vi "Drive Code.vi"() -> ()   [LabVIEW 2020]
uses:
  Team Code/Robot Global Data.vi
panel:
  out "LoopTime (ms)":u32
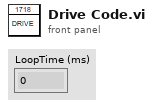
[diagram p1: front panel]
types:
  T1 = typedef "PiConfig.ctl" = cluster{"swerveModules":cluster{"leftFront":T2, "rightFront":T2, "leftRear":T2, "rightRear":T2}, "offsets":cluster{"leftFrontAngleOffset":dbl, "leftRearAngleOffset":dbl, "rightFrontAngleOffset":dbl, "rightRearAngleOffset":dbl}, "limits":cluster{"maxVelocity":dbl, "maxOverdriveVelocity":dbl, "maxAcceleration":dbl, "maxPickupVelocity":dbl, "maxClimbArmVelocity":dbl}, "speeds":cluster{"intakeSuckSpeed":dbl, "intakeSpitSpeed":dbl, "indexerSuckSpeed":dbl, "indexerSpitSpeed":dbl, "indexerShootSpeed":dbl, "indexerBumpBackSpeed":dbl, "shooterSpinupSpeed":dbl, "kickupSpinupSpeed":dbl, "shooterLowShootSpeed":dbl, "shooterHighShootSpeed":dbl, "shooterPadSpeed":dbl, "shooterWallSpeed":dbl}, "positions":cluster{"intakeStarting":dbl, "intakeStow":dbl, "intakeSuck":dbl, "armPounce":dbl, "armStow":dbl, "armUp":dbl, "winchPounce":dbl, "winchOut":dbl, "winchStow":dbl, "intakeSpit":dbl, "winchBarEngage":dbl, "winchBottomClimb":dbl, "hoodHighShoot":dbl, "armClearHooks":dbl, "winchClearHooks":dbl, "armLiftNextBar":dbl, "winchEngageHooksNextBar":dbl, "winchEngagePassive":dbl, "winchTraversalClimb":dbl, "hoodPadShoot":dbl, "turretPadShoot":dbl, "hoodWallShoot":dbl, "turretWallShoot":dbl, "winchRobotOffBar":dbl, "winchSettleClimb":dbl}, "inversions":cluster{"rightShooter":bool, "leftShooter":bool}}
  T2 = typedef "Swerve Module Parameters.ctl" = cluster{"driveCANID":dbl, "angleCANID":i32, "canCoderCANID":dbl, "moduleName":string, "driveMotorNeutralMode":T3, "driveCurrentLimitConfig":T4, "driveFeedbackDevice":T5, "driveInitialSensorPosition":dbl, "driveEnableVoltageComp":bool, "driveVoltageComp":dbl, "driveRampRate":dbl, "angleCurrentLimit":dbl, "angleSensorType":T6, "angleMotorType":T7, "angleConversionFactor":dbl, "anglePIDRamp":dbl, "angleVoltageComp":dbl, "angleIdleMode":T8, "cancoderConfig":T9, "angleInitialSensorPosition":dbl}
  T3 = typedef "CTRE_Phoenix_MotorControl_NeutralMode.ctl" = enum8{"EEPROMSetting", "Override to Coast", "Override to Brake"}
  T4 = typedef "CTRE_Phoenix_MotorControl_SupplyCurrentLimitConfiguration.ctl" = cluster{"Enable?":bool, "Current Limit":dbl, "Threshold Current":dbl, "Threshold Time":dbl}
  T5 = typedef "CTRE_Phoenix_MotorControl_FeedbackDevice_TalonFX.ctl" = i8
  T6 = typedef "Spark MAX Sensor Type.ctl" = enum16{"No Sensor", "Hall Sensor", "Encoder", "-Not Available-", "Analog", "Alternate Encoder"}
  T7 = typedef "Spark MAX Motor Type.ctl" = enum16{"Brushed", "Brushless"}
  T8 = typedef "Spark MAX Idle Mode.ctl" = enum16{"Coast", "Brake"}
  T9 = typedef "CTRE_Phoenix_CANcoder_Configurables.ctl" = cluster{"Sensor Initialization Strategy":T10, "Absolute Sensor Range":T11, "Velocity Measurement Period":T12, "Velocity Measurement Window":i32, "Magnet Offset (Degrees)":dbl, "Sensor Direction":bool, "Sensor Coefficient":dbl, "Unit String":string, "Sensor Time Base":T13}
  T10 = typedef "CTRE_Phoenix_CANcoder_SensorInitializationStrategy.ctl" = enum16{"Boot To Zero", "Boot To Absolute Position"}
  T11 = typedef "CTRE_Phoenix_CANcoder_AbsoluteSensorRange.ctl" = enum16{"Unsigned [0 to 360)", "Signed [-180 to +180)"}
  T12 = typedef "CTRE_Phoenix_MotorControl_VelocityMeasurementPeriod.ctl" = u16
  T13 = typedef "CTRE_Phoenix_CANcoder_SensorTimeBase.ctl" = enum16{"Per100Ms_Legacy", "PerSecond", "PerMinute"}
  T14 = typedef "Absolute Angle TypeDef.ctl" = cluster{"leftFrontAbsoluteAngle":dbl, "leftRearAbsoluteAngle":dbl, "rightFrontAbsoluteAngle":dbl, "rightRearAbsoluteAngle":dbl}
  T15 = cluster{"leftFrontDesiredVelocity":dbl, "leftRearDesiredVelocity":dbl, "rightFrontDesiredVelocity":dbl, "rightRearDesiredVelocity":dbl}
  T16 = cluster{"leftFrontSteeringPower":dbl, "leftRearSteeringPower":dbl, "rightFrontSteeringPower":dbl, "rightRearSteeringPower":dbl}
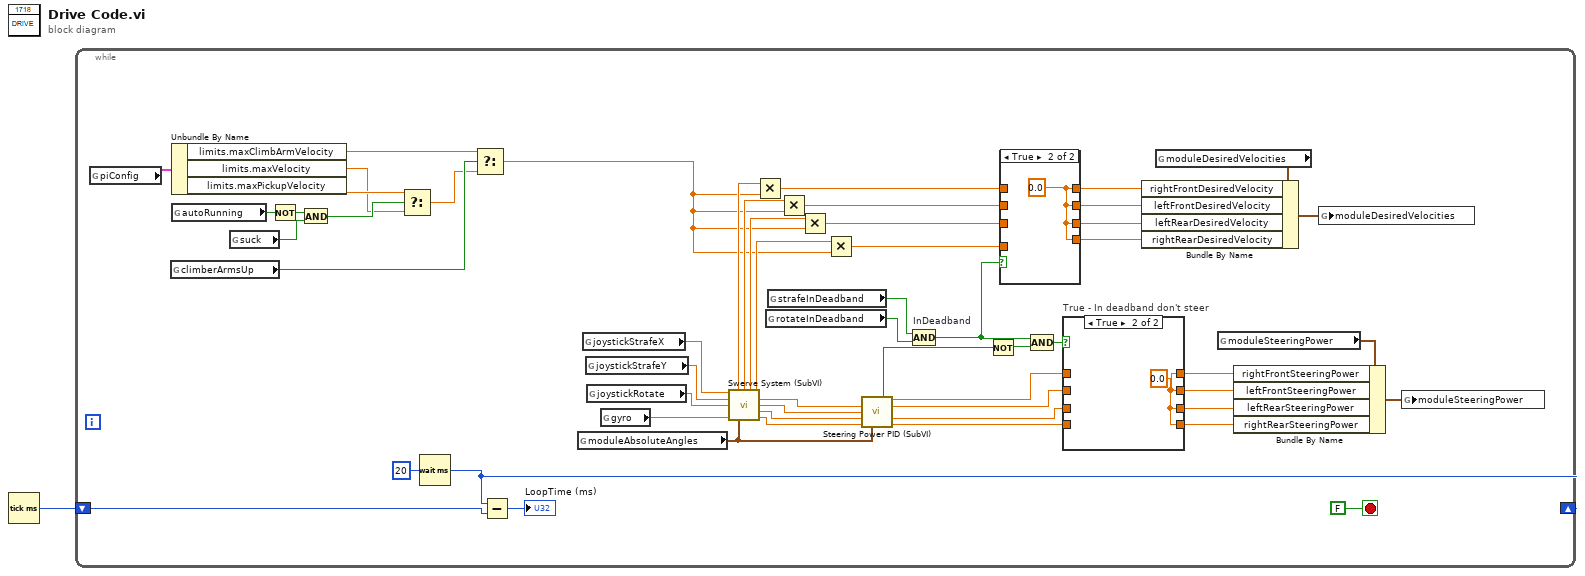
[diagram p0: block diagram]
diagram:
  n1 = Tick Count (ms)() -> (millisecond timer value=w1:u32)
  n2 = while {
    shift-right: [w39] -> _
    shift-left: w1 -> [w40]
    stop <- FALSE stop-if-true
    n3 = global read "Robot Global Data.vi" "piConfig"() -> (w48:T1)
    n4 = global read "Robot Global Data.vi" "climberArmsUp"() -> (w5:bool)
    n5 = Unbundle By Name(w48) -> ("limits.maxClimbArmVelocity"=w4:dbl, "limits.maxVelocity"=w6:dbl, "limits.maxPickupVelocity"=w7:dbl)
    n6 = global read "Robot Global Data.vi" "autoRunning"() -> (w14:bool)
    n7 = global read "Robot Global Data.vi" "suck"() -> (w36:bool)
    n8 = Not(x=w14) -> (.not. x?=w13:bool)
    n9 = And(x=w13, y=w36) -> (x .and. y?=w8:bool)
    n10 = Select(t=w7, s=w8, f=w6) -> (s? t:f=w3:dbl)
    n11 = Wait (ms)(milliseconds to wait=u32 20) -> (millisecond timer value=w39:u32)
    n12 = Select(t=w4, s=w5, f=w3) -> (s? t:f=w2:dbl)
    n13 = Subtract(x=w39, y=w40) -> (x-y=→"LoopTime (ms)":u32)
    n14 = global read "Robot Global Data.vi" "moduleAbsoluteAngles"() -> (w9:T14)
    n15 = global read "Robot Global Data.vi" "joystickStrafeX"() -> (w38:dbl)
    n16 = global read "Robot Global Data.vi" "joystickStrafeY"() -> (w37:dbl)
    n17 = global read "Robot Global Data.vi" "joystickRotate"() -> (w44:dbl)
    n18 = global read "Robot Global Data.vi" "gyro"() -> (w47:dbl)
    n19 = call "Swerve System (SubVI).vi"("Joystick 1 X (strafe)"=w38, "Joystick 1 Y (forward/back)"=w37, "Joystick 2 X (Rotate)"=w44, "Gyro Angle (deg)"=w47, "moduleAbsoluteAngles"=w9) -> ("RightFrontWheelPowerDesired"=w49:dbl, "LeftFrontWheelPowerDesired"=w50:dbl, "LeftRearWheelPowerDesired"=w51:dbl, "RightRearWheelPowerDesired"=w46:dbl, "rightFrontAngleError"=w19:dbl, "leftFrontAngleError"=w12:dbl, "leftRearAngleError"=w11:dbl, "rightRearAngleError"=w10:dbl)  [unwired: 3 in]
    n20 = Multiply(x=w49, y=w2) -> (x*y=w35:dbl)
    n21 = global read "Robot Global Data.vi" "rotateInDeadband"() -> (w43:bool)
    n22 = global read "Robot Global Data.vi" "strafeInDeadband"() -> (w56:bool)
    n23 = Multiply(x=w50, y=w2) -> (x*y=w34:dbl)
    n24 = Multiply(x=w51, y=w2) -> (x*y=w33:dbl)
    n25 = Multiply(x=w46, y=w2) -> (x*y=w32:dbl)
    n26 = call "Steering Power PID (SubVI).vi"("rightFrontAngleError"=w19, "leftFrontAngleError"=w12, "leftRearAngleError"=w11, "rightRearAngleError"=w10, "moduleAbsoluteAngles"=w9) -> ("overriden"=w26:bool, "rightFrontSteeringPower"=w18:dbl, "leftFrontSteeringPower"=w20:dbl, "leftRearSteeringPower"=w17:dbl, "rightRearSteeringPower"=w16:dbl)  [unwired: 6 in]
    n27 = Compound Arithmetic op=AND "InDeadband"(w56, w43) -> (w27:bool)
    n28 = Not(x=w26) -> (.not. x?=w25:bool)
    n29 = case shown="True" w27 {
      tunnel: w35 -> [w65 _]
      tunnel: w34 -> [w64 _]
      tunnel: w33 -> [w63 _]
      tunnel: w32 -> [w62 _]
      tunnel: [w65 w66] -> w31
      tunnel: [w64 w66] -> w30
      tunnel: [w63 w66] -> w29
      tunnel: [w62 w66] -> w28
      frame False {
      }
      frame True {
        w66 = 0.0
      }
    }
    n30 = Compound Arithmetic op=AND(w27, w25) -> (w15:bool)
    n31 = case "True - In deadband don't steer" shown="True" w15 {
      tunnel: w18 -> [w60 _]
      tunnel: [w60 w61] -> w24
      tunnel: [w58 w61] -> w23
      tunnel: [w57 w61] -> w22
      tunnel: [w59 w61] -> w21
      tunnel: w16 -> [w59 _]
      tunnel: w20 -> [w58 _]
      tunnel: w17 -> [w57 _]
      frame False {
      }
      frame True {
        w61 = 0.0 ("rightFrontSteeringPower")
      }
    }
    n32 = global read "Robot Global Data.vi" "moduleDesiredVelocities"() -> (w53:T15)
    n33 = Bundle By Name(cluster=w53, "rightFrontDesiredVelocity"=w31, "leftFrontDesiredVelocity"=w30, "leftRearDesiredVelocity"=w29, "rightRearDesiredVelocity"=w28) -> (w52:T15)
    n34 = global read "Robot Global Data.vi" "moduleSteeringPower"() -> (w54:T16)
    n35 = Bundle By Name(cluster=w54, "rightFrontSteeringPower"=w24, "leftFrontSteeringPower"=w23, "leftRearSteeringPower"=w22, "rightRearSteeringPower"=w21) -> (w55:T16)
    n36 = global write "Robot Global Data.vi" "moduleDesiredVelocities"(w52) -> ()
    n37 = global write "Robot Global Data.vi" "moduleSteeringPower"(w55) -> ()
  }
